vi "Set_Vi_Sate.vi"(9 "VI":refnum<vi>, 10 "Standard (T)":bool=TRUE, 11 "Activate (F)":bool) -> (1 "VI_out":refnum<vi>)   [LabVIEW 2019]
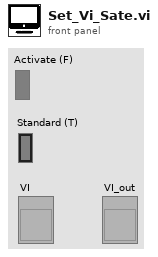
[diagram p1: front panel]
types:
  T1 = enum32{"Invalid", "Standard", "Closed", "Hidden", "Minimized", "Maximized"}
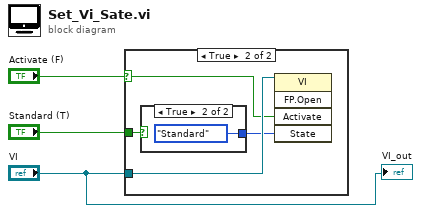
[diagram p0: block diagram]
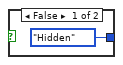
[diagram p3: hidden frame]
diagram:
  n1 = case shown="True" "Activate (F)" {
    selector: "Activate (F)" -> [_ w5]
    tunnel: "VI" -> [_ w7]
    tunnel: "Standard (T)" -> [_ w4]
    frame False {
    }
    frame True {
      n2 = case shown="True" w4 {
        tunnel: [T1."Hidden" ("State") T1."Standard" ("State")] -> w6
        frame False {
        }
        frame True {
        }
      }
      n3 = invoke class="VI" method="FP.Open"(reference=w7, "Activate"=w5, "State"=w6) -> ()  [unwired: 2 in, 5 out]
    }
  }
  "VI_out" <- "VI"
